vi "Remaining Duration.vi"(8 "error in (no error)":errorcluster, 9 "Remain Duration Data":T1 {"Total Duration" format="%#_8g"; "Cycle Duration" format="%#_8g"; "Running Cycle Number" format="%#_8g"; "Total Cycle Number" format="%#_8g"}, 10 "Schema":string, 11 "Auto UI in":refnum<class "Auto UI.lvclass">) -> (0 "error out":errorcluster, 3 "Auto UI out":refnum<class "Auto UI.lvclass">)   [LabVIEW 2023, in "GUI.lvlib" / "Auto UI.lvlib" / "Auto UI.lvclass"]
uses:
  Auto UI.lvclass
  Typdefs/Auto GUI/Remaining Duration.ctl
  Typdefs/Auto GUI/Duration.ctl
  Auto UI.lvclass/Auto UI.ctl
  Typdefs/Auto GUI/Test Info.ctl
  GUI.lvlib
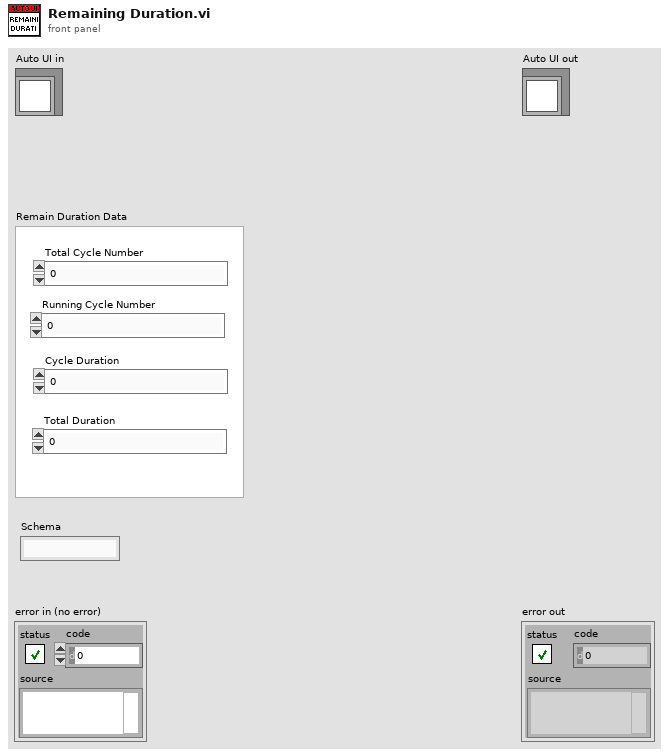
[diagram p1: front panel]
types:
  T1 = cluster{"Total Cycle Number":dbl, "Running Cycle Number":dbl, "Cycle Duration":dbl, "Total Duration":dbl}
  T2 = typedef "GUI.lvlib/Duration.ctl" = cluster{"Completed Duration":string, "Remaining Duration":string}
  T3 = typedef "GUI.lvlib/Remaining Duration.ctl" = cluster{"Hours":u8, "Min":u8, "Day":u8}
  T4 = typedef "GUI.lvlib/Test Info.ctl" = cluster{"Project Name":string, "Product Name":string, "Product Varient":string, "Test Name":string, "Test Start Time":string, "Estimated Date":string}
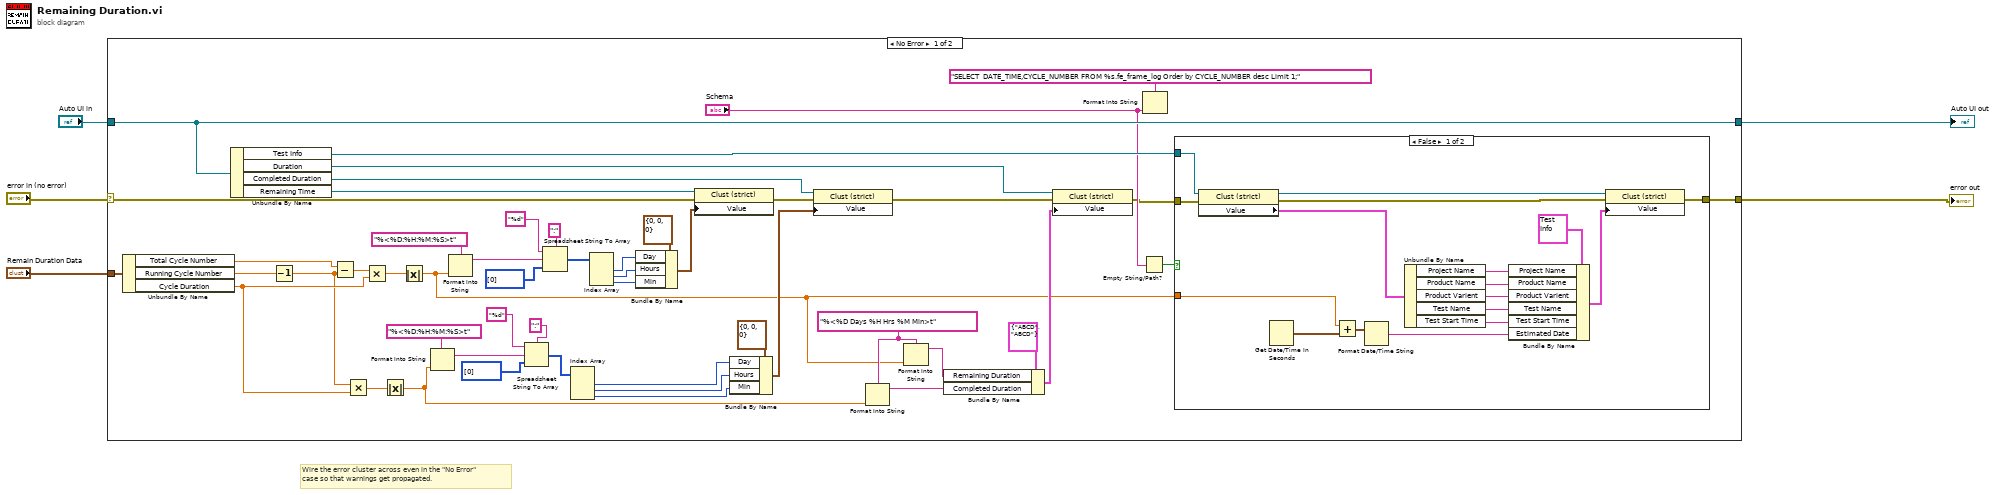
[diagram p0: block diagram]
diagram:
  # "Wire the error cluster across even in the \"No Error\"\ncase so that warnings get propagated."
  n1 = case shown="No Error" "error in (no error)" {
    selector: "error in (no error)" -> [w24 w75]
    tunnel: [w22 w75] -> w4
    tunnel: [w55 w74] -> w2
    tunnel: "Auto UI in" -> [w55 w74]
    tunnel: "Remain Duration Data" -> [w51 _]
    frame No Error {
      w9 = "%<%D Days %H Hrs %M Min>t" ("format string")
      n2 = Unbundle By Name(w51) -> ("Total Cycle Number"=w18:dbl, "Running Cycle Number"=w50:dbl, "Cycle Duration"=w20:dbl)
      n3 = Unbundle By Name(w55) -> ("Test Info"=w23:refnum<vi>, "Duration"=w15:refnum<vi>, "Completed Duration"=w38:refnum<vi>, "Remaining Time"=w54:refnum<vi>)
      n4 = Decrement(x=w50) -> (x-1=w19:dbl)
      n5 = Subtract(x=w18, y=w19) -> (x-y=w49:dbl)
      n6 = Multiply(x=w19, y=w20) -> (x*y=w37:dbl)
      n7 = Multiply(x=w49, y=w20) -> (x*y=w47:dbl)
      n8 = Absolute Value(x=w37) -> (abs(x)=w7:dbl)
      n9 = Absolute Value(x=w47) -> (abs(x)=w6:dbl)
      n10 = Format Into String(format string="%<%D:%H:%M:%S>t", w7) -> (resulting string=w36:string)  [unwired: 2 in, 1 out]
      n11 = Format Into String(format string="%<%D:%H:%M:%S>t", w6) -> (resulting string=w44:string)  [unwired: 2 in, 1 out]
      n12 = Spreadsheet String To Array(delimiter (Tab)=":", format string="%d", spreadsheet string=w36, array type (2D Dbl)=u8[] [0]) -> (array=w35:u8[])
      n13 = Spreadsheet String To Array(delimiter (Tab)=":", format string="%d", spreadsheet string=w44, array type (2D Dbl)=u8[] [0]) -> (array=w42:u8[])
      n14 = Index Array(array=w35) -> (element #1=w34:u8, element #2=w33:u8, element #3=w32:u8)  [unwired: 3 in]
      n15 = Index Array(array=w42) -> (element #1=w41:u8, element #2=w40:u8, element #3=w39:u8)  [unwired: 3 in]
      n16 = Bundle By Name(cluster=T3 {"Hours"=0, "Min"=0, "Day"=0} ("Value"), "Day"=w41, "Hours"=w40, "Min"=w39) -> (w52:T3)
      n17 = property class="Clust (strict)"(reference=w54, error in=w24, "Value"=w52) -> (error out=w25:errorcluster)  [unwired: 1 out]
      n18 = Bundle By Name(cluster=T3 {"Hours"=0, "Min"=0, "Day"=0} ("Value"), "Day"=w34, "Hours"=w33, "Min"=w32) -> (w26:T3)
      n19 = property class="Clust (strict)"(reference=w38, error in=w25, "Value"=w26) -> (error out=w14:errorcluster)  [unwired: 1 out]
      n20 = Format Into String(format string=w9, w7) -> (resulting string=w8:string)  [unwired: 2 in, 1 out]
      n21 = Format Into String(format string=w9, w6) -> (resulting string=w10:string)  [unwired: 2 in, 1 out]
      n22 = Bundle By Name(cluster=T2 {"Completed Duration"="ABCD", "Remaining Duration"="ABCD"} ("Value"), "Remaining Duration"=w10, "Completed Duration"=w8) -> (w11:T2)
      n23 = property class="Clust (strict)"(reference=w15, error in=w14, "Value"=w11) -> (error out=w13:errorcluster)  [unwired: 1 out]
      n24 = Empty String/Path?(string/path="Schema") -> (empty?=w17:bool)
      n25 = Format Into String(format string="SELECT  DATE_TIME,CYCLE_NUMBER FROM %s.fe_frame_log Order by CYCLE_NUMBER desc Limit 1;", "Schema") -> ()  [unwired: 2 in, 2 out]
      n26 = case shown="False" w17 {
        tunnel: w23 -> [w68 _]
        tunnel: [w72 w73] -> w22
        tunnel: w13 -> [w70 w73]
        tunnel: w6 -> [w56 _]
        frame False {
          n27 = property class="Clust (strict)"(reference=w68, error in=w70) -> (reference out=w67:refnum<vi>, error out=w69:errorcluster, "Value"=w64:T4)
          n28 = Get Date/Time In Seconds() -> (seconds since 1Jan1904=w57:timestamp)
          n29 = Add(x=w56, y=w57) -> (x+y=w71:timestamp)
          n30 = Format Date/Time String(seconds (now)=w71) -> (date/time string=w63:string)  [unwired: 2 in]
          n31 = Unbundle By Name(w64) -> ("Project Name"=w58:string, "Product Name"=w59:string, "Product Varient"=w60:string, "Test Name"=w61:string, "Test Start Time"=w62:string)
          n32 = Bundle By Name(cluster=T4 {"Project Name"="ABCD", "Product Name"="ABCD", "Product Varient"="ABCD", "Test Name"="ABCD", "Test Start Time"="ABCD", "Estimated Date"="ABCD"} ("Value"), "Project Name"=w58, "Product Name"=w59, "Product Varient"=w60, "Test Name"=w61, "Test Start Time"=w62, "Estimated Date"=w63) -> (w65:T4)
          n33 = property class="Clust (strict)"(reference=w67, error in=w69, "Value"=w65) -> (error out=w72:errorcluster)  [unwired: 1 out]
        }
        frame True {
        }
      }
    }
    frame Error {
    }
  }
  "error out" <- w4
  "Auto UI out" <- w2
